vi "Include_in_Build.vi"(8 "error in (no error)":errorcluster, 11 "AB_Source in":refnum<class "AB_Source.lvclass">) -> (0 "error out":errorcluster, 2 "includeInBuild":bool, 3 "AB_Source out":refnum<class "AB_Source.lvclass">)   [LabVIEW 2020, in "AB_Source.lvclass"]
uses:
  <vilib>/AppBuilder/AB_Classes/Source/AB_Source.lvclass
  <vilib>/AppBuilder/AB_Classes/Source/AB_Source.lvclass/AB_Source.ctl
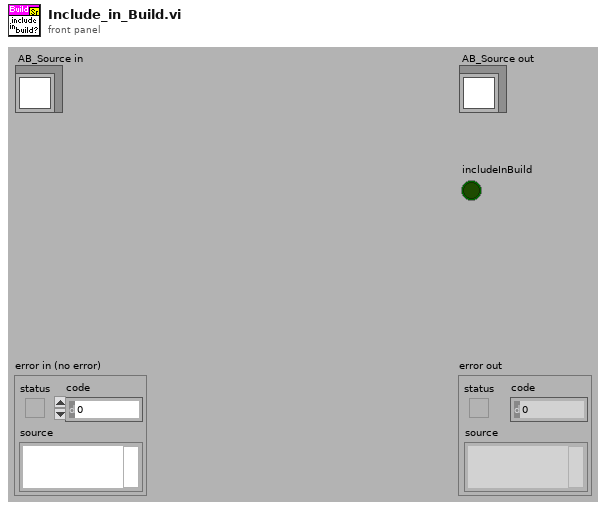
[diagram p1: front panel]
types:
  T1 = typedef "AB_Source_Inclusion.ctl" = enum16{"IncludeIfReferenced", "Include", "Exclude", "TopLevel"}
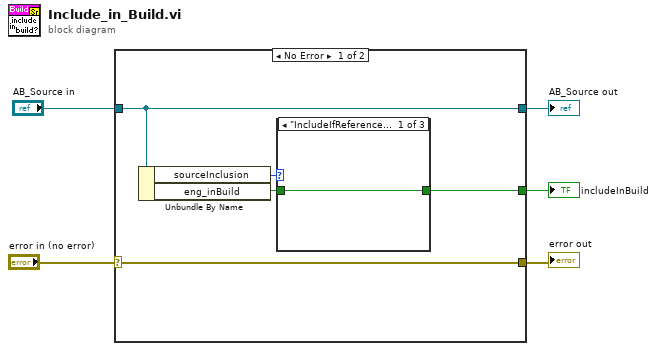
[diagram p0: block diagram]
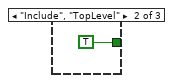
[diagram p2: hidden frame]
diagram:
  n1 = case shown="No Error" "error in (no error)" {
    selector: "error in (no error)" -> [w10 w14]
    tunnel: [w10 w14] -> w4
    tunnel: [w9 w13] -> w2
    tunnel: "AB_Source in" -> [w9 w13]
    tunnel: [w6 _] -> w1
    frame No Error {
      n2 = Unbundle By Name(w9) -> ("sourceInclusion"=w8:T1, "eng_inBuild"=w7:bool)
      n3 = case shown="\"IncludeIfReferenced\"" w8 {
        tunnel: [w11 TRUE ("eng_inBuild") _] -> w6
        tunnel: w7 -> [w11 _ _]
        frame "IncludeIfReferenced" {
        }
        frame "Include", "TopLevel" {
        }
        frame "Exclude" {
        }
      }
    }
    frame Error {
    }
  }
  "error out" <- w4
  "AB_Source out" <- w2
  "includeInBuild" <- w1
